vi "Act Measurements 2 Cart Measurements.vi"(3 "Type":T2=enum."X Actuators On The Left", 4 "LBCB Position":T1={"Motion Center"=[0.0, 0.0, 0.0], "Transformation Matrix"=[[1.0, 0.0, 0.0, 0.0, 0.0, 0.0], [0.0, 1.0, 0.0, 0.0, 0.0, 0.0], [0.0, 0.0, 1.0, 0.0, 0.0, 0.0], [0.0, 0.0, 0.0, 1.0, 0.0, 0.0], [0.0, 0.0, 0.0, 0.0, 1.0, 0.0], [0.0, 0.0, 0.0, 0.0, 0.0, 1.0]]}, 5 "Actuator Meas. \nDisp & Forces":dbl[](array[numeric])) -> (1 "Cart Measured\nDisp & Forces":dbl[](array[numeric]))   [LabVIEW 2009]
uses:
  Data Access Objects/Metadata/LBCB Type.ctl
  Data Access Objects/Metadata/LBCB Position.ctl
  LBCB_Conversions_Actions.ctl
panel:
  # "(inch)"
  # "X"
  # "(inch)"
  # "Y"
  # "(inch)"
  # "Z"
  # "Xglobal = T*Xlocal"
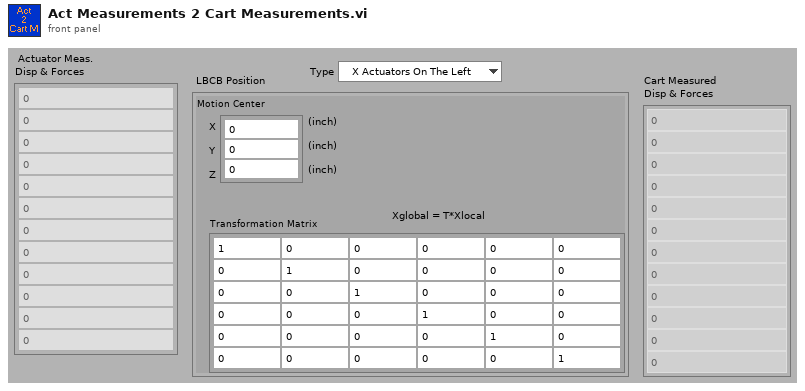
[diagram p1: front panel]
types:
  T1 = typedef "LBCB Position.ctl" = cluster{"Motion Center":dbl[], "Transformation Matrix":dbl[][]}
  T2 = typedef "LBCB Type.ctl" = enum16{"X Actuators On The Right", "X Actuators On The Left"}
  T3 = typedef "LBCB_Conversions_Actions.ctl" = enum16{"A2C", "C2A", "Set Log Filename", "Init"}
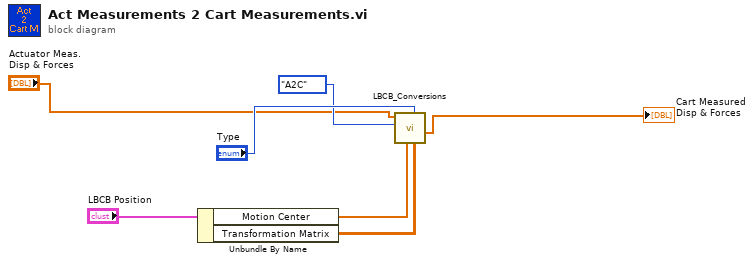
[diagram p0: block diagram]
diagram:
  n1 = Unbundle By Name("LBCB Position") -> ("Motion Center"=w4:dbl[], "Transformation Matrix"=w5:dbl[][])
  n2 = call "LBCB_Conversions.vi"("Transformation Matrix"=w5, "Type"="Type", "Motion Center"=w4, "Conversion Type"=LBCB_Conversions_Actions."A2C", "Input"="Actuator Meas. \nDisp & Forces") -> ("Output"=→"Cart Measured\nDisp & Forces":dbl[])  [unwired: 3 in, 3 out]
